vi "GoTo PID simples.vi"(8 "Position":dbl[](array[numeric]), 11 "Target":dbl[](array[numeric])) -> (3 "Velocity":dbl[](array[numeric]))   [LabVIEW 2016]
uses:
  <vilib>/Analysis/coordinate.llb/2D Cartesian Coordinate Rotation (Scalar).vi
  <vilib>/addons/control/pid/pid.llb/PID (DBL).vi
  <vilib>/addons/control/pid/NI_PID_pid.lvlib
  <vilib>/Analysis/NI_AALPro.lvlib
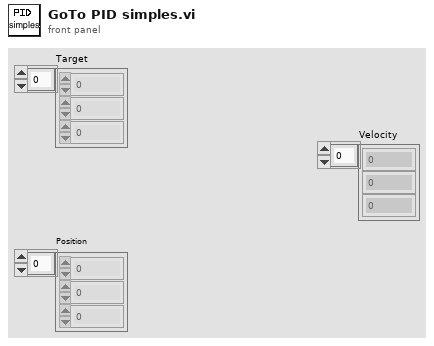
[diagram p1: front panel]
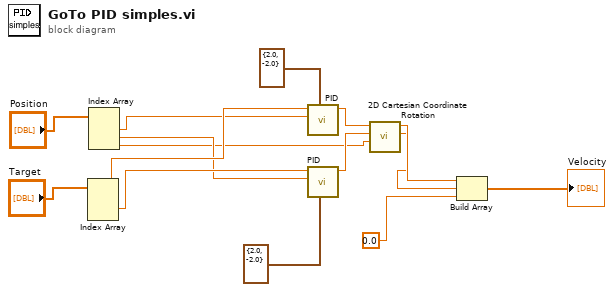
[diagram p0: block diagram]
diagram:
  n1 = Index Array(array="Target") -> (element #1=w12:dbl, element #2=w11:dbl)  [unwired: 3 in, 1 out]
  n2 = Index Array(array="Position") -> (element #1=w1:dbl, element #2=w10:dbl, element #3=w7:dbl)  [unwired: 3 in]
  n3 = call-poly <vilib>:"PID.vi"("output range"=cluster{"output high":dbl, "output low":dbl} {"output high"=2.0, "output low"=-2.0}, "process variable"=w1, "setpoint"=w12) -> ("output"=w9:dbl)  [unwired: 7 in, 1 out]
  n4 = call-poly <vilib>:"PID.vi"("output range"=cluster{"output high":dbl, "output low":dbl} {"output high"=2.0, "output low"=-2.0}, "process variable"=w10, "setpoint"=w11) -> ("output"=w8:dbl)  [unwired: 7 in, 1 out]
  n5 = call-poly <vilib>:"2D Cartesian Coordinate Rotation.vi"("theta"=w7, "y"=w8, "x"=w9) -> ("y out"=w5:dbl, "x out"=w6:dbl)  [unwired: 6 in, 1 out]
  n6 = Build Array(w6, w5, 0.0 ("element")) -> (→"Velocity":dbl[])
